vi "convertmm-to-psSD.vi"(1 "mm":dbl) -> (0 "ps":dbl)   [LabVIEW 2015]
uses:
  globalVarSD.vi
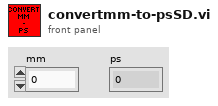
[diagram p1: front panel]
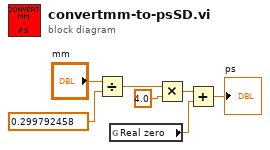
[diagram p0: block diagram]
diagram:
  n1 = Divide(x="mm", y=0.299792458) -> (x/y=w6:dbl)
  n2 = global read "globalVarSD.vi" "Real zero"() -> (w1:dbl)
  n3 = Multiply(x=w6, y=4.0) -> (x*y=w3:dbl)
  n4 = Add(x=w3, y=w1) -> (x+y=→"ps":dbl)
